vi "Get Module Identifiers.vi"(8 "error in":errorcluster, 11 "routing and faulting in":T1 format="%.0x") -> (0 "error out":errorcluster, 2 "module Identifier":string[](array[string]), 3 "routing and faulting out":T1 format="%.0x")   [LabVIEW 2017, in "Routing and Faulting Scripting.lvlib"]
uses:
  Routing and Faulting Scripting.lvlib
  <vilib>/NI Veristand/Custom Device API/Custom Device Item Ref.ctl
  NationalInstruments.VeriStand.SystemStorage
  Constants/Scripting Constants.vi
  <vilib>/NI Veristand/Custom Device API/Custom Device API.lvlib
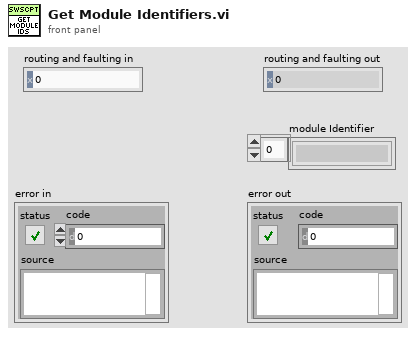
[diagram p1: front panel]
types:
  T1 = typedef "Custom Device API.lvlib/Custom Device Item Ref.ctl" = u64
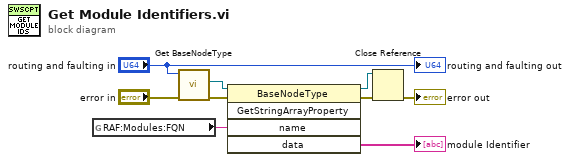
[diagram p0: block diagram]
diagram:
  n1 = global read "Scripting Constants.vi" "RAF:Modules:FQN"() -> (w9:string)
  n2 = call "Get BaseNodeType.vi"("error in (no error)"="error in", "Item Ref in"="routing and faulting in") -> ("error out"=w6:errorcluster, "BaseNodeType"=w5:refnum<k24>)  [unwired: 7 in, 1 out]
  n3 = invoke class="BaseNodeType" method="GetStringArrayProperty"(reference=w5, error in=w6, "name"=w9) -> (reference out=w2:refnum<k24>, error out=w4:errorcluster, "data"=→"module Identifier":string[])  [unwired: 2 in, 2 out]
  n4 = Close Reference(reference=w2, error in (no error)=w4) -> (error out=→"error out":errorcluster)
  "routing and faulting out" <- "routing and faulting in"
